vi "Prueba_PWM.vi"() -> ()   [LabVIEW 2025]
panel:
  in  "DC":u8(slide) scale=0.0..255.0
  in  "Pin":u8=4 min=4 max=40
  in  "VISA resource name":refnum<visa-resource-name>
  in  "stop":bool
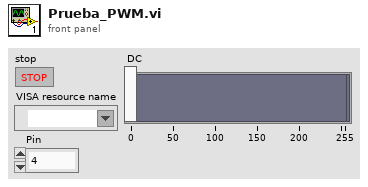
[diagram p1: front panel]
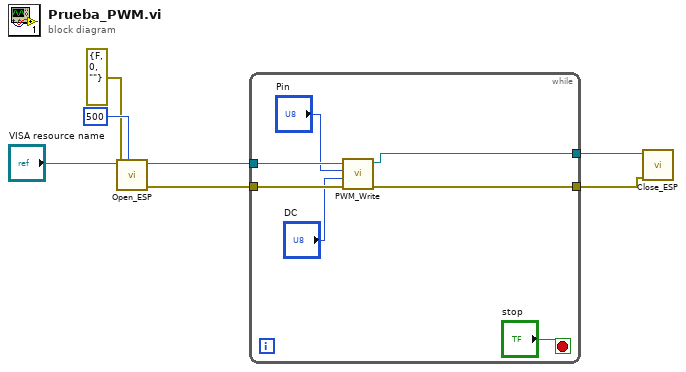
[diagram p0: block diagram]
diagram:
  n1 = call "Open_ESP.vi"("timeout (10sec)"=u32 500, "error in (no error)"=errorcluster {"status"=FALSE, "code"=0, "source"=""}, "VISA resource name"="VISA resource name") -> ("error out"=w5:errorcluster, "VISA resource name out"=w4:refnum<visa-resource-name>)  [unwired: 7 in]
  n2 = while {
    tunnel: [w13] -> w7
    tunnel: [w12] -> w6
    tunnel: w5 -> [w11]
    tunnel: w4 -> [w10]
    stop <- "stop" stop-if-true
    n3 = call "PWM_Write.vi"("error in (no error)"=w11, "DC"="DC", "Pin"="Pin", "VISA resource name"=w10) -> ("error out"=w12:errorcluster, "VISA resource name out"=w13:refnum<visa-resource-name>)  [unwired: 6 in]
  }
  n4 = call "Close_ESP.vi"("error in (no error)"=w6, "VISA resource name"=w7) -> ()  [unwired: 9 in, 1 out]
